vi "Upgrade Addon to Latest Version.vi"(8 "error in (no error)":errorcluster, 11 "Device Item Ref in in":T1 format="%.0x") -> (0 "error out":errorcluster, 3 "Device Item Ref out":T1 format="%.0x")   [LabVIEW 2019, in "Control Addon System Explorer.lvlib"]
uses:
  Control Addon System Explorer.lvlib
  NationalInstruments.VeriStand.SystemDefinitionAPI
  <vilib>/NI VeriStand/Custom Device API/Custom Device API.lvlib
  Shared/Constants.vi
  Shared/Control Addon Shared.lvlib
  <vilib>/NI VeriStand/Custom Device API/Custom Device Item Ref.ctl
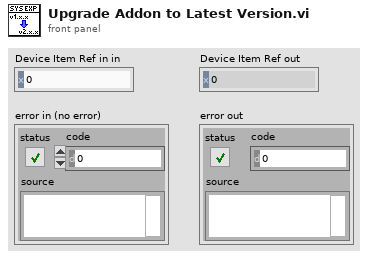
[diagram p1: front panel]
types:
  T1 = typedef "Custom Device API.lvlib/Custom Device Item Ref.ctl" = u64
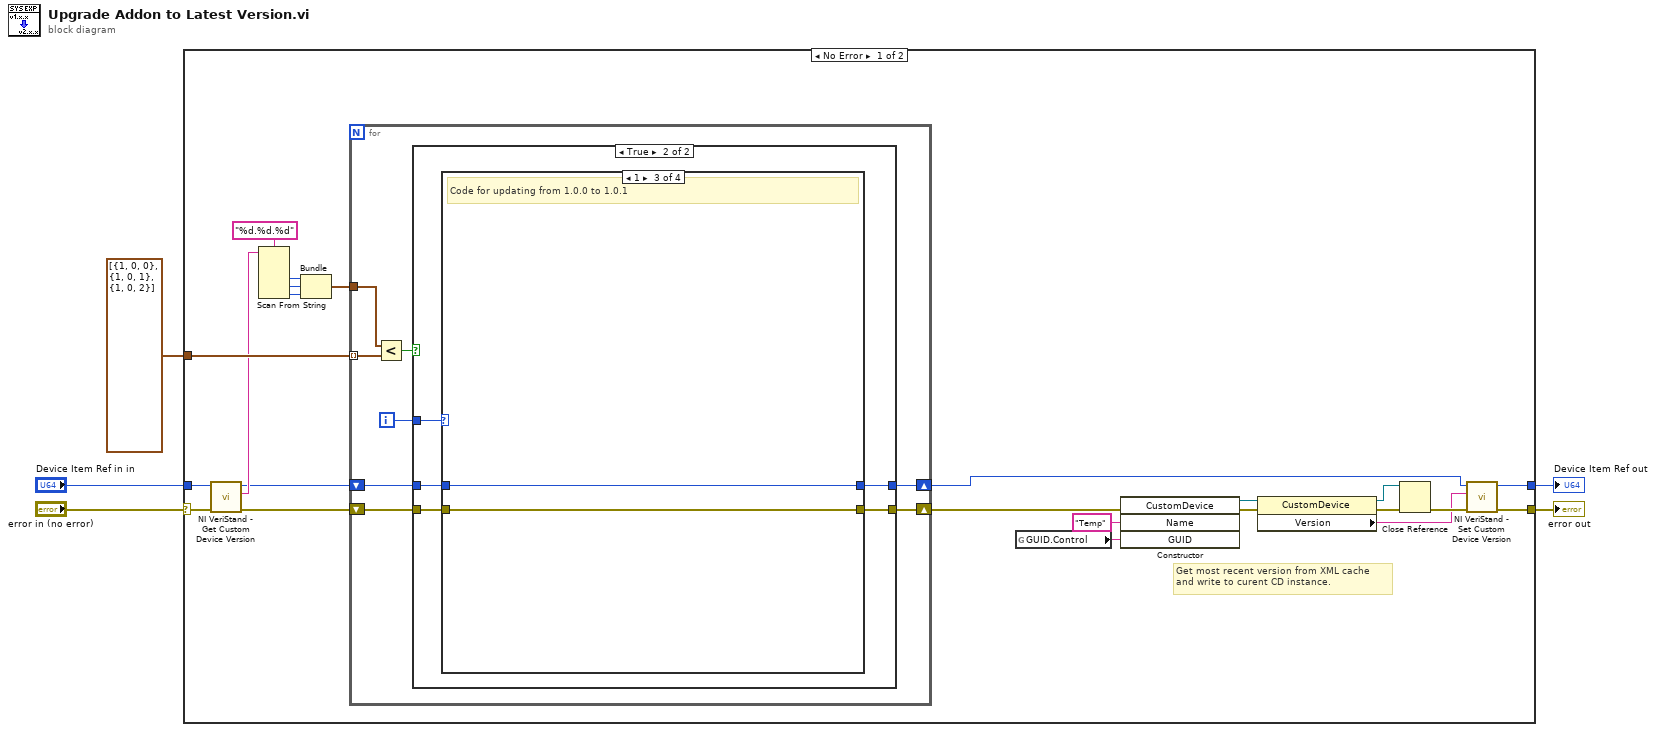
[diagram p0: block diagram]
diagram:
  n1 = case shown="No Error" "error in (no error)" {
    selector: "error in (no error)" -> [w12 w53]
    tunnel: [w21 w53] -> w4
    tunnel: "Device Item Ref in in" -> [w11 w52]
    tunnel: [w20 w52] -> w5
    tunnel: cluster{i32, i32, i32}[] [{1, 0, 0}, {1, 0, 1}, {1, 0, 2}] -> [w28 _]
    frame No Error {
      # "Get most recent version from XML cache\nand write to curent CD instance."
      n2 = call <vilib>:"NI VeriStand - Get Custom Device Version.vi"("error in (no error)"=w12, "Device Ref in"=w11) -> ("error out"=w8:errorcluster, "Value"=w16:string, "Device Ref out"=w7:T1)  [unwired: 7 in]
      n3 = Scan From String(format string="%d.%d.%d", input string=w16) -> (output 1=w14:i32, output 2=w13:i32, output 3=w15:i32)  [unwired: 5 in, 3 out]
      n4 = Bundle(w14, w13, w15) -> (w9:cluster{i32, i32, i32})  [unwired: 1 in]
      n5 = for {
        tunnel: w28 -> [w34] mode=indexing
        shift-right: [w36] -> w19
        shift-left: w8 -> [w30]
        shift-right: [w35] -> w18
        shift-left: w7 -> [w29]
        tunnel: w9 -> [w31]
        i -> [w32]
        n6 = Less?(x=w31, y=w34) -> (x < y?=w33:bool)
        n7 = case shown="True" w33 {
          tunnel: w30 -> [w38 w43]
          tunnel: [w38 w42] -> w36
          tunnel: w29 -> [w37 w39]
          tunnel: [w37 w40] -> w35
          tunnel: w32 -> [_ w41]
          frame False {
          }
          frame True {
            n8 = case shown="1" w41 {
              tunnel: w43 -> [w45 w47 w49 w51]
              tunnel: [w45 w47 w49 w51] -> w42
              tunnel: [w44 w46 w48 w50] -> w40
              tunnel: w39 -> [w44 w46 w48 w50]
              frame Default {
                # "Nothing to update"
              }
              frame 0 {
                # "Initial Onload"
              }
              frame 1 {
                # "Code for updating from 1.0.0 to 1.0.1"
              }
              frame 2 {
                # "Code for updating from 1.0.1 to 1.0.2"
              }
            }
          }
        }
      }
      n9 = global read "Constants.vi" "GUID.Control"() -> (w6:string)
      n10 = constructor class="CustomDevice"(error in=w19, "Name"="Temp", "GUID"=w6) -> (reference out=w27:refnum<k24>, error out=w26:errorcluster)  [unwired: 2 in, 3 out]
      n11 = property class="CustomDevice"(reference=w27, error in=w26) -> (reference out=w24:refnum<k24>, error out=w25:errorcluster, "Version"=w22:string)
      n12 = Close Reference(reference=w24, error in (no error)=w25) -> (error out=w23:errorcluster)
      n13 = call <vilib>:"NI VeriStand - Set Custom Device Version.vi"("error in (no error)"=w23, "Value"=w22, "Device Ref in"=w18) -> ("error out"=w21:errorcluster, "Device Ref out"=w20:T1)  [unwired: 7 in]
    }
    frame Error {
    }
  }
  "Device Item Ref out" <- w5
  "error out" <- w4
